vi "Split Event Name.vi"(11 "Event Name":string) -> (1 "Lvlib?":bool, 2 "Vi Name":string, 3 "Library Name":string)   [LabVIEW 2021, in "TAF Proj Document Type.lvlib"]
uses:
  <vilib>/Wovalab/AntiDoc/Document Type/Add-ons/LabVIEW TAF Project/TAF Proj Document Type.lvlib
  <vilib>/Wovalab/AntiDoc/Utilities/Utilities.lvlib
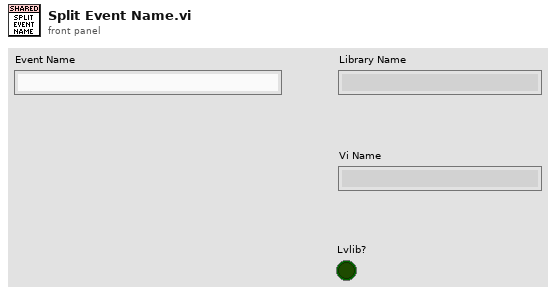
[diagram p1: front panel]
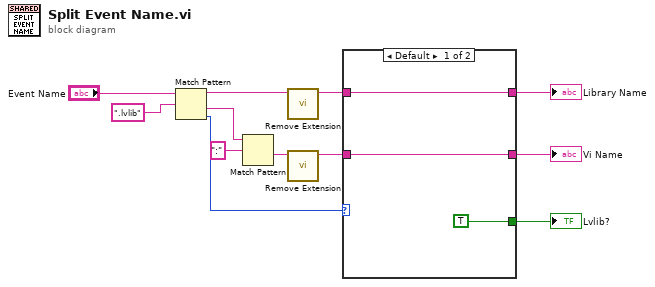
[diagram p0: block diagram]
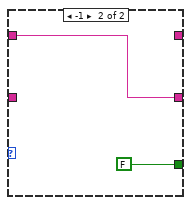
[diagram p2: hidden frame]
diagram:
  n1 = Match Pattern(string="Event Name", regular expression=".lvlib") -> (before substring=w4:string, after substring=w5:string, offset past match=w10:i32)  [unwired: 1 in, 1 out]
  n2 = Match Pattern(string=w5, regular expression=":") -> (after substring=w2:string)  [unwired: 1 in, 3 out]
  n3 = call <vilib>:"Remove Extension.vi"("File Name"=w4) -> ("File Name Without Extension"=w3:string)  [unwired: 10 in]
  n4 = call <vilib>:"Remove Extension.vi"("File Name"=w2) -> ("File Name Without Extension"=w1:string)  [unwired: 10 in]
  n5 = case shown="Default" w10 {
    tunnel: w3 -> [w15 w16]
    tunnel: w1 -> [w14 _]
    tunnel: [w15 _] -> w9
    tunnel: [w14 w16] -> w8
    tunnel: [TRUE FALSE] -> w7
    frame Default {
    }
    frame -1 {
    }
  }
  "Vi Name" <- w8
  "Library Name" <- w9
  "Lvlib?" <- w7
